vi "BaseGui.vi"() -> ()   [LabVIEW 2016]
uses:
  BaseGui.Action.ctl
  tools/CitTemplate/citTemplate.errData.ctl
  tools/EventLog/EventLog.EventSource.ctl
  <vilib>/Utility/miscctls.llb/LVRowAndColumnUnsignedTypeDef.ctl
  <vilib>/Utility/miscctls.llb/LVRowAndColumnTypeDef.ctl
  Station/Station.State.ctl
  Sequence/Sequence.MainMode.ctl
  Global/ApplicationGlobal.vi
  Station/Station.Global.vi
  Sequence/Sequence.Global.vi
panel:
  out "Progress":bool
  out "_loop":i32(ring)=4
  out "Gui open":bool
  out "Panel":refnum<vi>
  in  "StartHere...":bool
  out "StatusTable":i32(listbox)
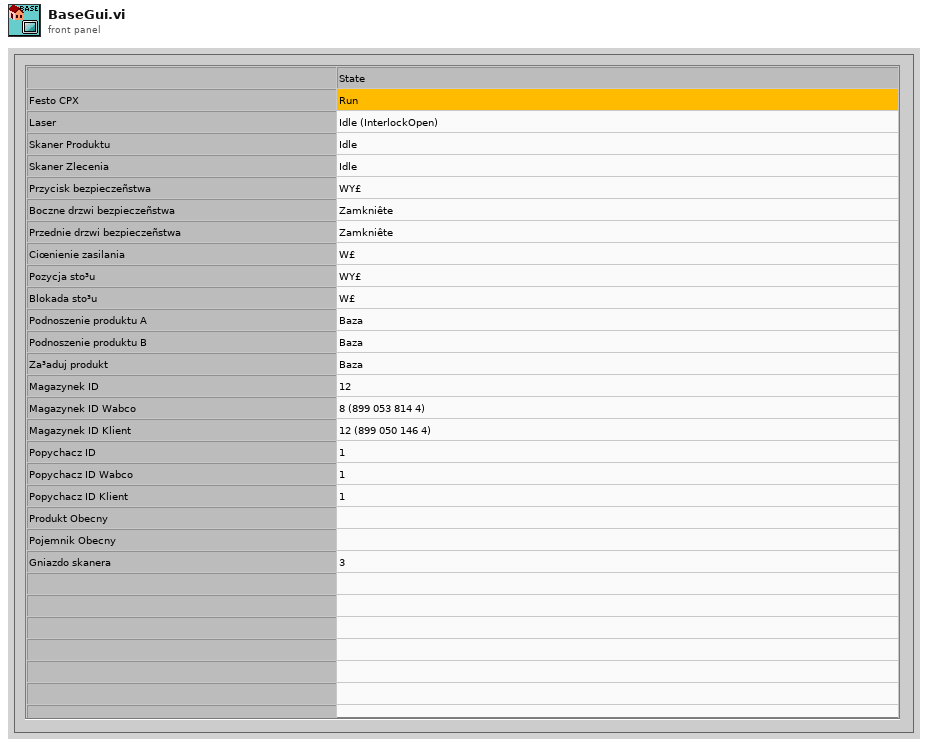
[diagram p1: front panel]
types:
  T1 = typedef "BaseGui.Action.ctl" = enum32{"idle", "constructor", "destructor", "--- BaseGui ---", "Status.Update", "Home.Done"}
  T2 = typedef "citTemplate.errData.ctl" = cluster{"ts":timestamp, "src":T3, "instance":i32, "action":string, "error":errorcluster, "unconfirmed":bool}
  T3 = typedef "EventLog.EventSource.ctl" = enum16{"All", "Gui", "Ref", "File", "Arch", "Seq", "CPX", "DB", "Laser", "Scan.P", "Scan.O"}
  T4 = enum8{"Enabled", "Disabled", "Disabled and Grayed Out"}
  T5 = typedef "Station.State.ctl" = enum16{"Idle", "Ready", "Run", "Stop", "Error", "Home", "Done", "Emg"}
  T6 = typedef "LVRowAndColumnTypeDef.ctl" = cluster{"Row":i32, "Column":i32}
  T7 = typedef "LVRowAndColumnUnsignedTypeDef.ctl" = cluster{"Row":u32, "Column":u32}
  T8 = typedef "Sequence.MainMode.ctl" = enum16{"Process", "Base", "Order", "Manual", "Logs", "Results", "Stats", "DMC Config"}
  T9 = typedef "citTemplate.notifierHandle.ctl" = refnum<notifier>
  T10 = enum32{"Invalid", "Standard", "Closed", "Hidden", "Minimized", "Maximized"}
  T11 = typedef "LVPositionTypeDef.ctl" = cluster{"Left":i32, "Top":i32}
  T12 = typedef "Station.Home.Status.ctl" = cluster{"status":bool, "color":u32, "msg":string}
  T13 = typedef "Station.Data.ctl" = cluster{"State":T5, "Seq.State":T14, "Seq.BreakReason":T15, "Seq.BreakSource":T16, "Hw failure":bool, "Unconfirmed":bool, "Station empty":bool, "Home err":bool, "Order done":bool, "DUT present":T17, "EmgState":T18, "Sets":T19, "StatusBits":T21}
  T14 = typedef "Sequence.State.ctl" = enum16{"Init", "Idle", "Home", "Work", "Run", "Pause"}
  T15 = typedef "Sequence.Test.BreakReason.ctl" = enum16{"-", "NOK container", "OK container", "Rev empty", "Rev missing", "Rev wrong", "Fork missing", "Fork wrong", "NOK limit", "Unload failure", "Single slot", "Part done", "Err: Prod move work", "Err: Prod move home", "Err: Prod lift work", "Err: Prod lift home", "Err: Prod Arm Work", "Err: Prod Arm NOK", "Err: Prod Arm OK", "Err: Prod NOK suck", "Err: Prod NOK drop", "Err: Prod OK missing", "Err: Prod OK suck", "Err: Prod OK drop"}
  T16 = typedef "Sequence.Test.BreakSource.ctl" = enum16{"-", "A", "B", "A/B"}
  T17 = typedef "FestoCPX.Station.ProdPresent.ctl" = cluster{"Slot1":cluster{"A":bool, "B":bool}, "Slot2":cluster{"A":bool, "B":bool}, "Slot3":cluster{"A":bool, "B":bool}, "Slot4":cluster{"A":bool, "B":bool}, "Final":cluster{"A":bool, "B":bool}, "OK":cluster{"A":bool, "B":bool}, "Container":cluster{"OK":bool, "NOK":bool}}
  T18 = typedef "FestoCPX.Station.EmgState.ctl" = cluster{"Button":bool, "SideDoor":bool, "FrontDoor":bool, "DoorSecured":bool}
  T19 = typedef "Sequence.UserData.ctl" = cluster{"GuiMode":T8, "Test":T20, "ContinueOrder":bool}
  T20 = typedef "MainGui.TestOptions.ctl" = cluster{"IgnoreResults":bool, "IgnoreImages":bool, "ServiceMode":bool}
  T21 = typedef "Station.Home.Status.Bits.ctl" = cluster{"Door Close":bool, "Rev OK":bool, "Fork OK":bool, "Container OK":bool, "Station empty":bool}
  T22 = typedef "Sequence.Data.ctl" = cluster{"BeginTS":timestamp, "EndTS":timestamp, "State":T14, "Status.Work":T23, "Status.Process":T23, "Status.Home":T23, "Status.Wabco":T23, "Status.Client":T23, "BreakReason":T15, "BreakSource":T16, "DoorLock":bool, "Status.Prod":T24[], "UserAction":T28, "UserData":T19, "Error":errorcluster, "Code":T29, "Rotations":i32, "ProdIdx":i32, "ProdDone":T24[], "PrintedSerials-Wabco":i32[], "PrintedSerials-Client":i32[], "Counters-Wabco":T36, "Counters-Client":T36}
  T23 = typedef "Sequence.Step.Status.ctl" = enum16{"-", "Pending", "Running", "Skipped", "Passed", "Failed", "Done", "Error", "Aborted", "Stopped"}
  T24 = typedef "Sequence.Test.Status.ctl" = cluster{"Slot":T25, "A":T27, "B":T27}
  T25 = typedef "Sequence.Slot.StatusData.ctl" = cluster{"ID":i32, "Unload":T26, "TS":timestamp, "duration":u32}
  T26 = typedef "Sequence.Test.Unload.Status.ctl" = enum16{"init", "check NOK", "check OK", "wait on NOK", "wait on OK", "wait on Unload", "done"}
  T27 = typedef "Sequence.Prod.StatusData.ctl" = cluster{"status":T23, "pause":T15, "present":bool, "printed":bool, "scanned":bool, "tuned":bool, "removed":bool, "LaserVariables":string[], "Serial":i32, "ScannerReadOut":string, "path":path, "corners":cluster{"X":i32, "Y":i32}[], "verification":u8}
  T28 = typedef "Sequence.UserActions.ctl" = cluster{"Stop":bool, "Pause":bool, "Next":bool}
  T29 = typedef "Sequence.Code.Sets.ctl" = cluster{"Ready":bool, "DoubleOrder":bool, "OrderDone":bool, "AllowSingleSlot":bool, "CheckDM":bool, "ThresholdA":u8, "ThresholdB":u8, "Plate":T30, "ImgPath":path, "Variant":T31}
  T30 = typedef "Sequence.PlateType.ctl" = enum16{"Wabco", "Client"}
  T31 = typedef "Logger.Variant.Sets.ctl" = cluster{"State":T32, "ImgPath":path, "WabcoPlate":string, "WabcoProduct":string, "ClientProduct":string, "ClientPlate":string, "TotalQuantity":u16, "OrderQuantity":u16, "Serial":i32, "Wabco":T33, "Client":T33}
  T32 = typedef "Station.Changeover.State.vi" = enum16{"Init", "Scaning", "NOK", "Wait for ack", "Ready"}
  T33 = typedef "Station.Plate.Properties.ctl" = cluster{"LaserJob":string, "AdditionalTxt":string, "FactoryCode":string, "RevID":u8, "ForkID":u8, "FailuresLimit":u16, "GlobalCnt":i32, "ScannerProgram":u8, "SerialFormat":T34, "CoordA":T35, "CoordB":T35, "DMCconfig":i32, "CVX_Program":u16}
  T34 = typedef "Sequence.Code.SerialFormat.ctl" = enum8{"", "6 dig", "7 dig"}
  T35 = typedef "V7310.Job.Sets.ctl" = cluster{"X":dbl, "Y":dbl, "Angle":dbl}
  T36 = typedef "Sequence.Counters.ctl" = cluster{"Expected":u16, "Done":u16, "OK":u16, "NOK":u16, "NOKlimit":u16, "Part":u16, "PartOK":u16}
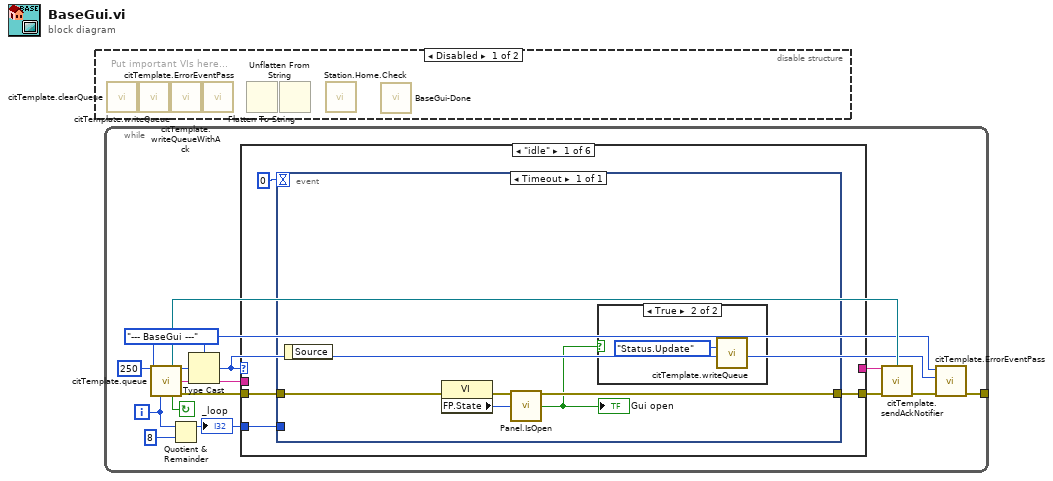
[diagram p0: block diagram]
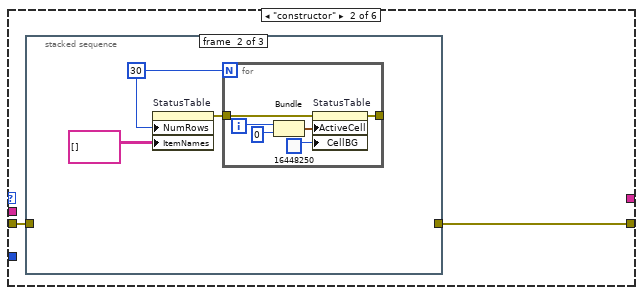
[diagram p3: hidden frame]
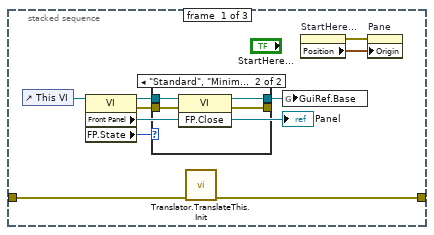
[diagram p4: hidden frame]
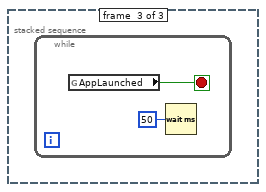
[diagram p6: hidden frame]
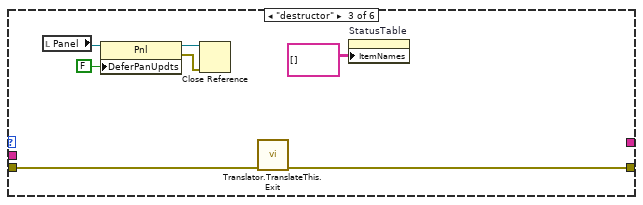
[diagram p7: hidden frame]
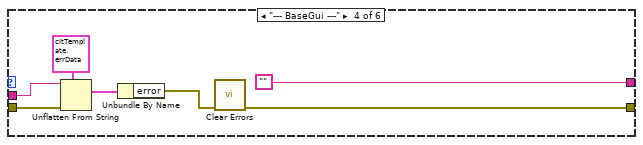
[diagram p8: hidden frame]
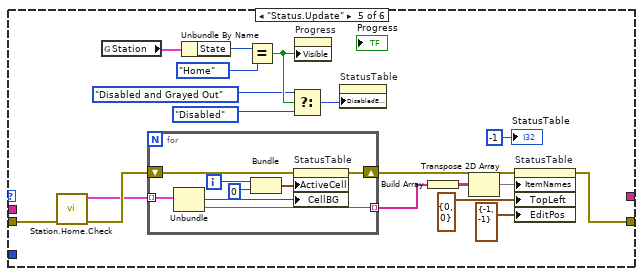
[diagram p9: hidden frame]
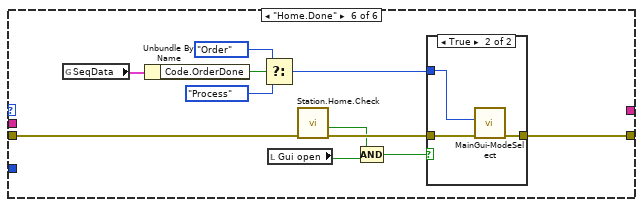
[diagram p10: hidden frame]
diagram:
  n1 = disable-structure shown="Disabled" {
    frame Disabled {
      # "Put important VIs here..."
      n2 = call "citTemplate.clearQueue.vi"() -> ()  [unwired: 14 in, 2 out]
      n3 = call "citTemplate.writeQueue.vi"() -> ()  [unwired: 15 in, 1 out]
      n4 = call "citTemplate.writeQueueWithAck.vi"() -> ()  [unwired: 13 in, 3 out]
      n5 = call "citTemplate.ErrorEventPass.vi"() -> ()  [unwired: 11 in, 1 out]
      n6 = Flatten To String() -> ()  [unwired: 4 in, 3 out]
      n7 = Unflatten From String() -> ()  [unwired: 5 in, 3 out]
      n8 = call "Station.Home.Check.vi"() -> ()  [unwired: 7 in, 5 out]
      n9 = call "BaseGui-Done.vi"() -> ()  [unwired: 11 in, 1 out]
    }
    frame Enabled {
    }
  }
  n10 = while {
    tunnel: [w3] -> _
    i -> [w5]
    stop <- w11 continue-if-true
    w8 = BaseGui.Action."--- BaseGui ---" ("Action")
    n11 = call "citTemplate.queue.vi"("ms timeout (250 ms)"=250, "event enum"=w8, "iteration (-1)"=w5) -> ("notifierHandle out"=w10:T9, "event out"=w14:u32, "(flatten) data out"=w13:string, "continue"=w11:bool, "error out"=w12:errorcluster)  [unwired: 2 in, 6 out]
    n12 = Quotient & Remainder(x=w5, y=8) -> (x-y*floor(x/y)=w1:i32)  [unwired: 1 out]
    "_loop" <- w1
    n13 = Type Cast(type=w8, x=w14) -> (*(type *) &x=w4:T1)
    n14 = case shown="\"idle\"" w4 {
      tunnel: w13 -> [_ _ _ w65 _ _]
      tunnel: w12 -> [w17 w24 w58 w63 w75 w101]
      tunnel: [_ _ _ "" _ _] -> w9
      tunnel: [w16 w25 w59 w64 w74 w103] -> w7
      tunnel: w1 -> [w15 _ _ _ _ _]
      frame "idle" {
        n15 = event shown="[0] Timeout" {
          selector: _ -> [_]
          dyn-events: _ -> [_]
          timeout: 0 -> [_]
          tunnel: w17 -> [w22]
          tunnel: [w21] -> w16
          tunnel: w15 -> [_]
          event Timeout {
            n16 = event-data() -> ()  [unwired: 1 in, 1 out]
            n17 = property class="VI"(error in=w22) -> (error out=w21:errorcluster, "FP.State"=w20:T10)  [unwired: 1 in, 1 out]
            n18 = call "Panel.IsOpen.vi"("FP State"=w20) -> ("Open?"=w19:bool)
            "Gui open" <- w19
            n19 = case shown="True" w19 {
              frame False {
              }
              frame True {
                n20 = call "citTemplate.writeQueue.vi"("event in (if not connected:all statemachine with data event)"=BaseGui.Action."Status.Update" ("Action")) -> ()  [unwired: 14 in, 1 out]
              }
            }
          }
        }
      }
      frame "constructor" {
        n21 = stacked-sequence {
          tunnel: [w30 _ _] -> w25
          tunnel: w24 -> [w31 _ _]
          frame #0 {
            n22 = control-ref of="This VI"() -> (w32:refnum<vi>)
            n23 = property class="VI"(reference=w32) -> (reference out=w29:refnum<vi>, error out=w28:errorcluster, "Front Panel"=→"Panel":refnum<vi>, "FP.State"=w27:T10)  [unwired: 1 in]
            n24 = case shown="\"Standard\", \"Minimized\", \"Maximized\"" w27 {
              tunnel: w29 -> [w37 w41]
              tunnel: w28 -> [w36 w40]
              tunnel: [w37 w39] -> w26
              tunnel: [w36 w38] -> _
              frame Default {
              }
              frame "Standard", "Minimized", "Maximized" {
                n25 = invoke class="VI" method="FP.Close"(reference=w41, error in=w40) -> (reference out=w39:refnum<vi>, error out=w38:errorcluster)  [unwired: 1 in, 1 out]
              }
            }
            n26 = call "Translator.TranslateThis.Init.vi"("error in"=w31) -> ("error out"=w30:errorcluster)  [unwired: 10 in]
            n27 = global write "ApplicationGlobal.vi" "GuiRef.Base"(w26) -> ()
            n28 = property on="StartHere..." class="Bool (strict)"() -> (error out=w34:errorcluster, "Position"=w33:T11)  [unwired: 2 in, 1 out]
            n29 = property on="Pane" class="Pane"(error in=w34, "Origin"=w33) -> ()  [unwired: 1 in, 2 out]
          }
          frame #1 {
            w44 = 30
            n30 = property on="StatusTable" class="MCListbox (strict)"("NumRows"=w44, "ItemNames"=string[][] [] ("Item Names")) -> (error out=w43:errorcluster)  [unwired: 2 in, 1 out]
            n31 = for {
              N: w44 -> [_]
              tunnel: [w46] -> _
              tunnel: w43 -> [w45]
              i -> [w48]
              n32 = Bundle(w48, 0) -> (w49:cluster{i32, i32})  [unwired: 1 in]
              n33 = property on="StatusTable" class="MCListbox (strict)"(error in=w45, "ActiveCell"=w49, "CellBG"=u32 16448250) -> (error out=w46:errorcluster)  [unwired: 1 in, 1 out]
            }
          }
          frame #2 {
            n34 = while {
              stop <- w52 stop-if-true
              n35 = global read "ApplicationGlobal.vi" "AppLaunched"() -> (w52:bool)
              n36 = Wait (ms)(milliseconds to wait=u32 50) -> ()  [unwired: 1 out]
            }
          }
        }
      }
      frame "destructor" {
        n37 = local read "Panel"() -> (w53:refnum<vi>)
        n38 = property class="Pnl"(reference=w53, "DeferPanUpdts"=FALSE ("Defer Panel Updates")) -> (reference out=w55:refnum<vi>, error out=w56:errorcluster)  [unwired: 1 in]
        n39 = Close Reference(reference=w55, error in (no error)=w56) -> ()  [unwired: 1 out]
        n40 = call "Translator.TranslateThis.Exit.vi"("error in"=w58) -> ("error out"=w59:errorcluster)  [unwired: 10 in]
        n41 = property on="StatusTable" class="MCListbox (strict)"("ItemNames"=string[][] [] ("Item Names")) -> ()  [unwired: 2 in, 2 out]
      }
      frame "--- BaseGui ---" {
        n42 = Unflatten From String(type=T2 {"ts"=timestamp(0 s since 1904-01-01), "src"=enum."All", "instance"=0, "action"="", "error"={"status"=FALSE, "code"=0, "source"=""}, "unconfirmed"=FALSE} ("ErrData"), binary string=w65, error in (no error)=w63) -> (value=w61:T2)  [unwired: 4 out]
        n43 = Unbundle By Name(w61) -> ("error"=w60:errorcluster)
        n44 = call <vilib>:"Clear Errors.vi"("error in (no error)"=w60) -> ("error out"=w64:errorcluster)  [unwired: 5 in, 1 out]
      }
      frame "Status.Update" {
        n45 = call "Station.Home.Check.vi"("error in (no error)"=w75) -> ("error out"=w77:errorcluster, "Statuses"=w76:T12[])  [unwired: 6 in, 3 out]
        n46 = global read "Station.Global.vi" "Station"() -> (w73:T13)
        n47 = for {
          tunnel: w76 -> [w88] mode=indexing
          shift-right: [w90] -> w81
          shift-left: w77 -> [w86]
          tunnel: [w85] -> w80 mode=indexing
          i -> [w89]
          n48 = Unbundle(w88) -> ("color"=w87:u32, "msg"=w85:string)  [unwired: 1 out]
          n49 = Bundle(w89, 0) -> (w92:cluster{i32, i32})  [unwired: 1 in]
          n50 = property on="StatusTable" class="MCListbox (strict)"(error in=w86, "ActiveCell"=w92, "CellBG"=w87) -> (error out=w90:errorcluster)  [unwired: 1 in, 1 out]
        }
        n51 = Unbundle By Name(w73) -> ("State"=w72:T5)
        n52 = Equal?(x=w72, y=Station.State."Home") -> (x = y?=w70:bool)
        n53 = Select(t=T4."Disabled and Grayed Out" ("Disabled"), s=w70, f=T4."Disabled" ("Disabled")) -> (s? t:f=w67:T4)
        n54 = property on="Progress" class="Bool (strict)"("Visible"=w70) -> ()  [unwired: 2 in, 2 out]
        n55 = property on="StatusTable" class="MCListbox (strict)"("DisabledEnum"=w67) -> ()  [unwired: 2 in, 2 out]
        n56 = Build Array(w80) -> (w79:string[][])
        n57 = Transpose 2D Array(2D array=w79) -> (transposed array=w78:string[][])
        n58 = property on="StatusTable" class="MCListbox (strict)"(error in=w81, "ItemNames"=w78, "TopLeft"=T7 {"Row"=0, "Column"=0} ("Top Left Visible Cell"), "EditPos"=T6 {"Row"=-1, "Column"=-1} ("Edit Position")) -> (error out=w74:errorcluster)  [unwired: 1 in, 1 out]
        "StatusTable" <- -1 ("Status")
      }
      frame "Home.Done" {
        n59 = global read "Sequence.Global.vi" "SeqData"() -> (w97:T22)
        n60 = Unbundle By Name(w97) -> ("Code.OrderDone"=w96:bool)
        n61 = Select(t=Sequence.MainMode."Order" ("Mode"), s=w96, f=Sequence.MainMode."Process" ("Mode")) -> (s? t:f=w93:T8)
        n62 = local read "Gui open"() -> (w102:bool)
        n63 = call "Station.Home.Check.vi"("error in (no error)"=w101) -> ("error out"=w100:errorcluster, "Homed?"=w98:bool)  [unwired: 6 in, 3 out]
        n64 = Compound Arithmetic op=AND(w98, w102) -> (w99:bool)
        n65 = case shown="True" w99 {
          tunnel: [w104 w107] -> w103
          tunnel: w100 -> [w104 w106]
          tunnel: w93 -> [_ w105]
          frame False {
          }
          frame True {
            n66 = call "MainGui-ModeSelect.vi"("error in (no error)"=w106, "Mode"=w105) -> ("error out"=w107:errorcluster)  [unwired: 9 in]
          }
        }
      }
    }
    n67 = call "citTemplate.sendAckNotifier.vi"("notification data"=w9, "notifierHandle in"=w10, "error in"=w7) -> ()  [unwired: 13 out]
    n68 = call "citTemplate.ErrorEventPass.vi"("error in"=w7, "action of error"=w4, "event in"=w8) -> ("error out"=w3:errorcluster)  [unwired: 2 in, 6 out]
  }
